vi "api_mqttDisconnect.vi"(11 "error in (no error)":errorcluster) -> (4 "success":bool, 15 "error out":errorcluster)   [LabVIEW 2018, in "mqtt.lvclass"]
uses:
  mqtt.lvclass
  mqttTypedef/mqttQOSlevel.ctl
  mqttTypedef/mqttMessageType.ctl
  mqttCmd/mqttCmdDisconnect/mqttCmdDisconnect.lvclass
  mqttCmd/mqttCmd.lvclass/mqttCmd.ctl
  mqttCmd/mqttCmd.lvclass
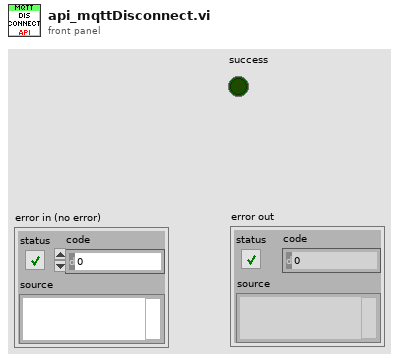
[diagram p1: front panel]
types:
  T1 = typedef "mqttMessageType.ctl" = enum32{"Reserved", "CONNECT", "CONNACK", "PUBLISH", "PUBACK", "PUBREC", "PUBREL", "PUBCOMP", "SUBSCRIBE", "SUBACK", "UNSUBSCRIBE", "UNSUBACK", "PINGREQ", "PINGRESP", "DISCONNECT", "Reserved2"}
  T2 = typedef "mqttQOSlevel.ctl" = enum8{"At most once", "At least once", "Exactly once", "Reserved"}
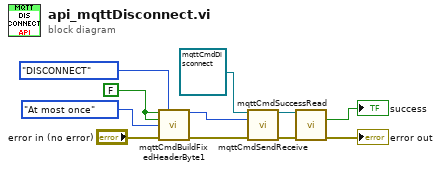
[diagram p0: block diagram]
diagram:
  w8 = FALSE
  n1 = call "mqttCmdBuildFixedHeaderByte1.vi"("retain(F)"=w8, "MessageType"=mqttMessageType."DISCONNECT", "duplicate(F)"=w8, "QoS (At most once)"=mqttQOSlevel."At most once", "error in (no error)"="error in (no error)") -> ("byte1"=w10:u8, "error out"=w6:errorcluster)  [unwired: 9 in]
  n2 = call "mqttCmdSendReceive.vi"("mqttConnect in"=refnum<class "mqttCmdDisconnect.lvclass"> refnum ("mqttBrokerCommandDisconnect.lvclass"), "byte1"=w10, "error in (no error)"=w6) -> ("mqttConnect out"=w4:refnum<class "mqttCmdDisconnect.lvclass">, "error out"=w5:errorcluster)  [unwired: 10 in, 1 out]
  n3 = call "mqttCmdSuccessRead.vi"("mqttBrokerCommand in"=w4, "error in (no error)"=w5) -> ("success"=→"success":bool, "error out"=→"error out":errorcluster)  [unwired: 11 in, 1 out]
